vi "V to mV (waveform).vi"(8 "Boolean":bool, 11 "input signal":waveform(dbl)) -> (3 "output":waveform(dbl))   [LabVIEW 2020]
doc: "Converts input signal (waveform) in volts to millivolts if Boolean input returns TRUE. Otherwise, data flows unchanged"
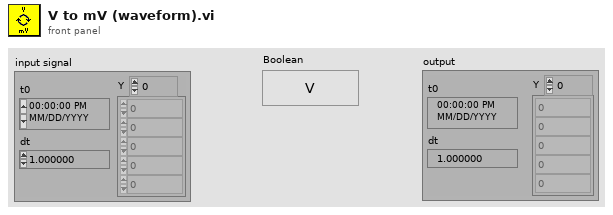
[diagram p1: front panel]
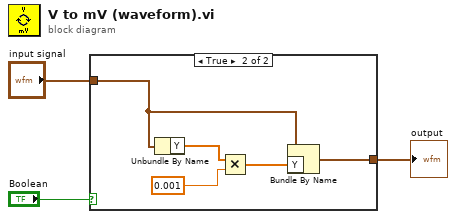
[diagram p0: block diagram]
diagram:
  n1 = case shown="True" "Boolean" {
    tunnel: "input signal" -> [w4 w6]
    tunnel: [w4 w5] -> w2
    frame False {
    }
    frame True {
      n2 = Unbundle By Name(w6) -> ("Y"=w9:dbl[])
      n3 = Multiply(x=w9, y=0.001) -> (x*y=w7:dbl[])
      n4 = Bundle By Name(cluster=w6, "Y"=w7) -> (w5:waveform(dbl))
    }
  }
  "output" <- w2
